vi "Axsun_module.vi"() -> ()   [LabVIEW 2018]
uses:
  cluster_Axsun.ctl
  Queue Manager Actions.ctl
  MessagePacket.ctl
  QueueNames.ctl
  D:/serial sectioning OCT/Axsun laser/AxsunOCTControlConsoleApplicationProject/AxsunOCTControlConsoleApplicationProject/AxsunOCTControl.dll
  AxsunOCTControlConsoleApplicationProject/AxsunOCTControlConsoleApplicationProject/AxsunOCTControl.dll
panel:
  in  "clock delay":u32
  in  "GetStatus":bool
  in  "LaserOnTime":bool
  out "output cluster":T1
  out "GUI error":errorcluster
  in  "Source current OFF":bool
  in  "Source current ON":bool
  in  "stop":bool
  in  "Laser OFF":bool
  in  "Laser ON":bool
  out "processor error":errorcluster
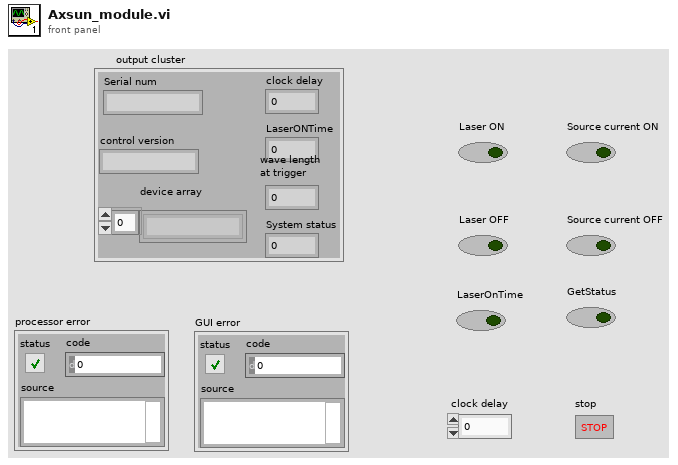
[diagram p1: front panel]
types:
  T1 = typedef "cluster_Axsun.ctl" = cluster{"device array":string[], "control version":string, "Serial num":string, "LaserONTime":i32, "wave length\nat trigger":dbl, "System status":dbl, "clock delay":u32}
  T2 = typedef "MessagePacket.ctl" = cluster{"Message":string, "Parameter":variant}
  T3 = typedef "Queue Manager Actions.ctl" = enum16{"Init", "Enqueue", "Enqueue All", "Preview Queue", "Dequeue", "Get Status", "Flush Queue", "Flush All Queues", "Release All Queues", "Release Queue", "Enqueue at Opposite End"}
  T4 = typedef "QueueNames.ctl" = enum16{"Main GUI", "Main Scan Processor", "Axsun GUI", "Axsun processor", "Main Display", "Main Table Stage GUI", "Main Table Stage Proc.", "Scan Engine", "Vibratome GUI", "Vibratome Processor", "Slice Engine"}
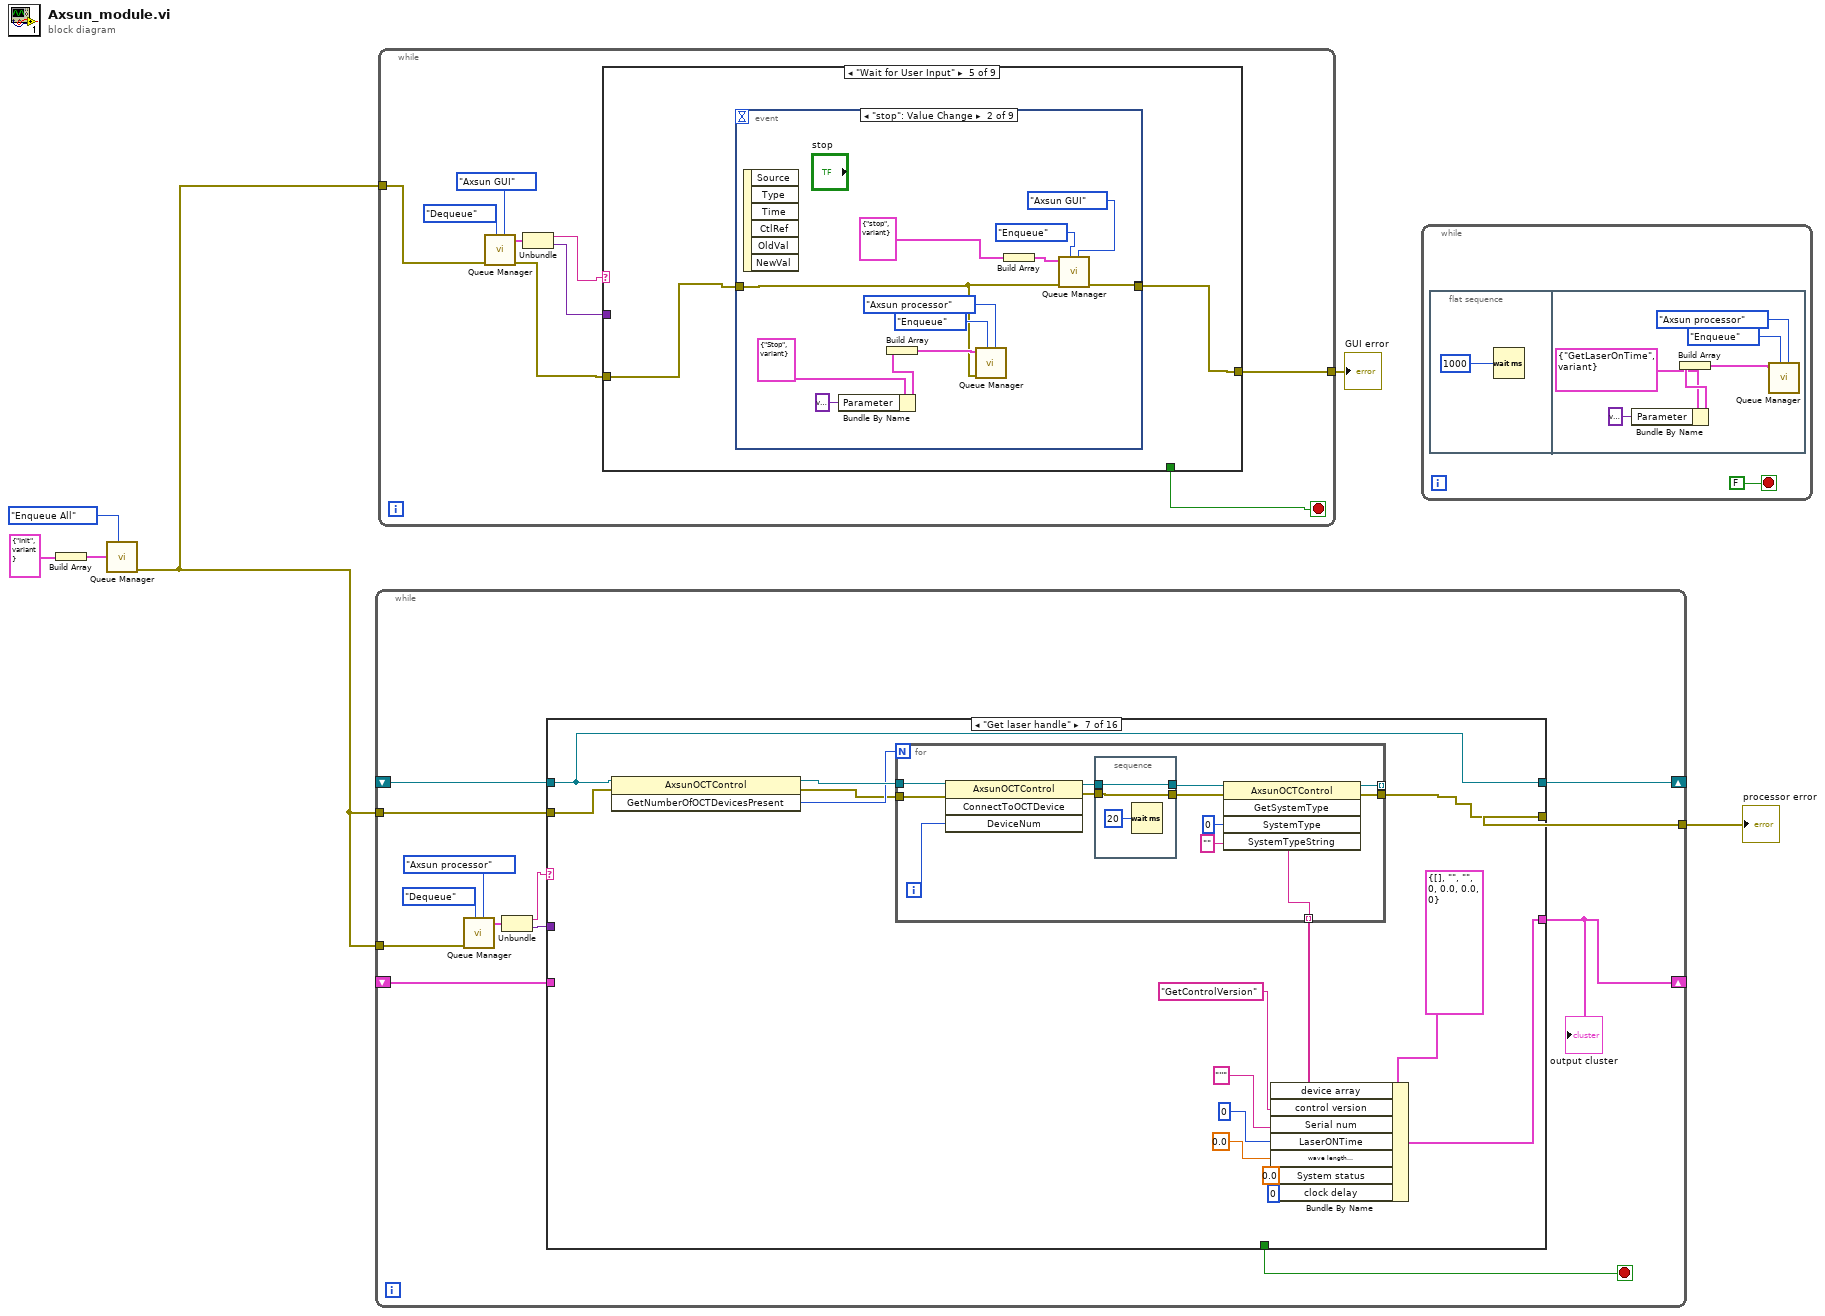
[diagram p0: block diagram]
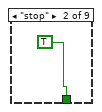
[diagram p3: hidden frame]
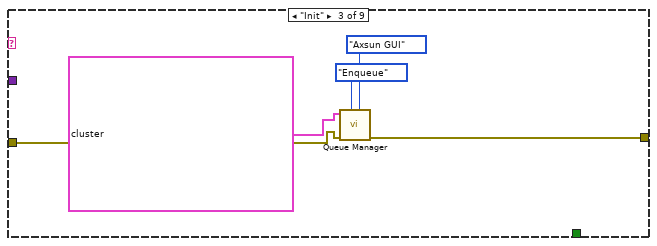
[diagram p4: hidden frame]
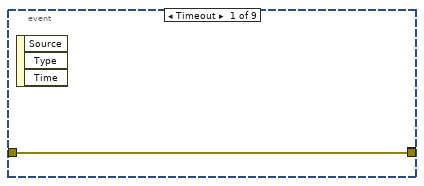
[diagram p6: hidden frame]
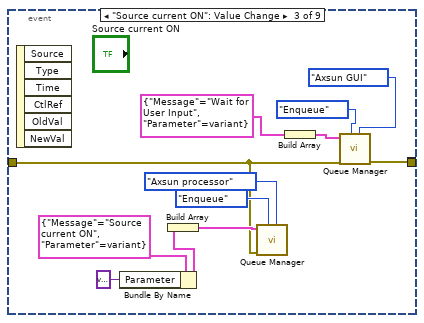
[diagram p7: hidden frame]
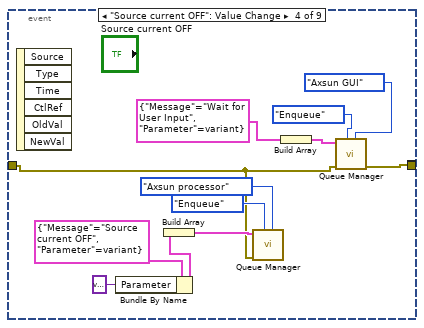
[diagram p8: hidden frame]
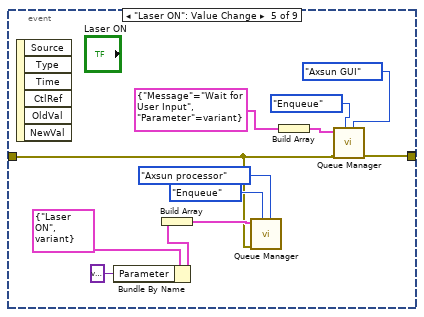
[diagram p9: hidden frame]
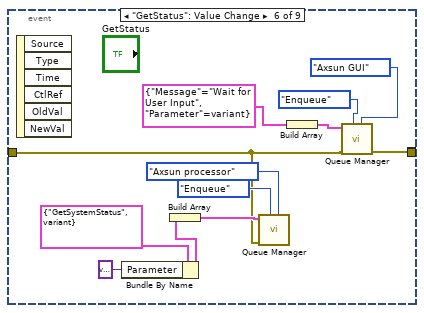
[diagram p10: hidden frame]
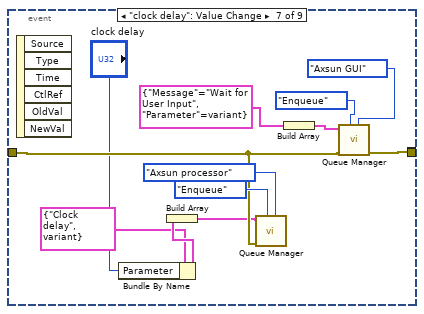
[diagram p11: hidden frame]
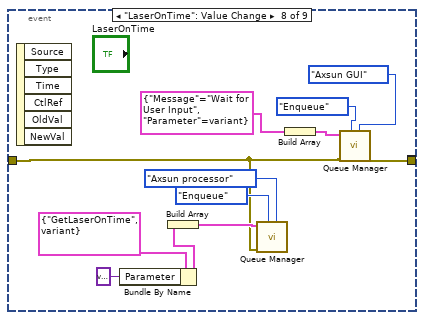
[diagram p12: hidden frame]
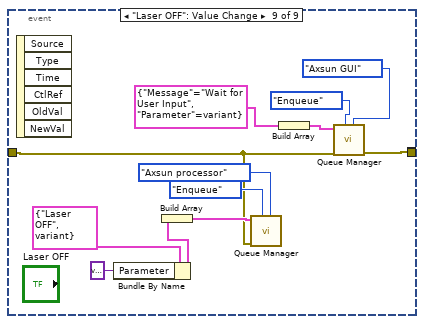
[diagram p13: hidden frame]
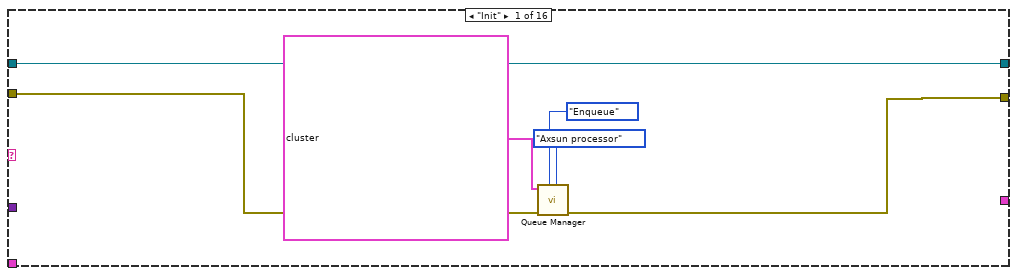
[diagram p18: hidden frame]
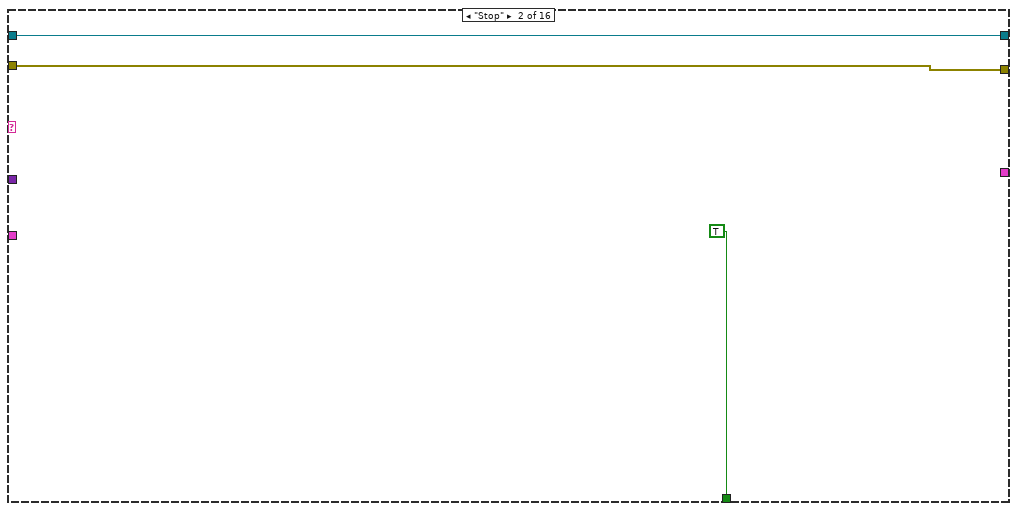
[diagram p19: hidden frame]
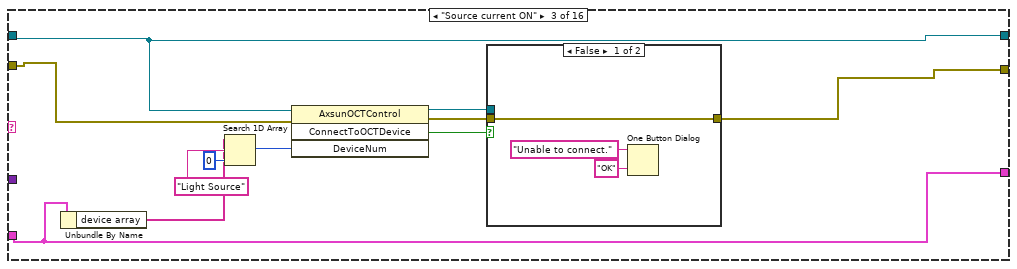
[diagram p20: hidden frame]
diagram:
  n1 = Build Array(T2 {"Message"="Init", "Parameter"=variant} ("Message Packet [In]")) -> (w4:T2[])
  n2 = call "Queue Manager.vi"("Action"=Queue_Manager_Actions."Enqueue All", "Message Packet Array"=w4) -> ("Error Out"=w2:errorcluster)  [unwired: 7 in, 2 out]
  n3 = while {
    shift-right: [w13] -> _
    shift-left: _ -> [w12]
    tunnel: w2 -> [w15]
    shift-right: [w7] -> _
    shift-left: _ -> [w10]
    tunnel: [w9] -> w3
    tunnel: w2 -> [w8]
    stop <- w14 stop-if-true
    n4 = call "Queue Manager.vi"("Queue Name"=QueueNames."Axsun processor", "Action"=Queue_Manager_Actions."Dequeue", "Error In"=w8) -> ("Message Packet [Out]"=w17:T2)  [unwired: 6 in, 2 out]
    n5 = Unbundle(w17) -> ("Message"=w11:string, "Parameter"=w16:variant)
    n6 = case shown="\"Get laser handle\"" w11 {
      tunnel: w16 -> [_ _ _ _ _ _ _ _ _ _ w170 _ _ _ _ _]
      tunnel: w15 -> [w25 w27 w33 w49 w65 w70 w88 w108 w126 w148 w171 w200 w218 w225 w246 _]
      tunnel: [_ TRUE _ _ _ _ _ _ _ _ _ _ _ _ _ _] -> w14
      tunnel: [w20 w26 w31 w48 w64 w67 w83 w106 w127 w146 w167 w198 w216 w226 _ w265] -> w13
      tunnel: w12 -> [w20 w26 w31 w48 w64 w71 w83 w106 w127 w146 w167 w198 w219 w226 w247 _]
      tunnel: [w21 w27 w32 w50 w65 w68 w84 w107 w125 w147 w166 w199 w217 w224 w245 w264] -> w9
      tunnel: [_ _ w30 w47 w63 w66 w76 w105 w124 w144 w164 w197 w214 w220 w241 w263] -> w7
      tunnel: w10 -> [_ _ w30 w47 w63 w66 _ w105 w122 w143 w165 w197 w215 w222 w243 w263]
      frame "Init" {
        n7 = call "Queue Manager.vi"("Queue Name"=QueueNames."Axsun processor", "Action"=Queue_Manager_Actions."Enqueue", "Error In"=w25, "Message Packet Array"=T2[] [{"Message"="Create handle", "Parameter"=variant}, {"Message"="Start Network Control Interface", "Parameter"=variant}, {"Message"="Get laser handle", "Parameter"=variant}, {"Message"="GetControlVersion", "Parameter"=variant}, {"Message"="GetSerialNum", "Parameter"=variant}, {"Message"="GetSystemStatus", "Parameter"=variant}, {"Message"="GetWaveLengthAtSweptTrigger", "Parameter"=variant}, {"Message"="GetLaserOnTime\nGetLaserOnTime", "Parameter"=variant}]) -> ("Error Out"=w21:errorcluster)  [unwired: 5 in, 2 out]
      }
      frame "Stop" {
      }
      frame "Source current ON" {
        n8 = Unbundle By Name(w30) -> ("device array"=w29:string[])
        n9 = Search 1D Array(1D array=w29, element="Light Source", start index (0)=0) -> (index of element=w37:i32)
        n10 = invoke class="AxsunOCTControl" method="ConnectToOCTDevice"(reference=w31, error in=w33, "DeviceNum"=w37) -> (reference out=w36:refnum<k24>, error out=w35:errorcluster, "ConnectToOCTDevice"=w34:bool)  [unwired: 1 in, 1 out]
        n11 = case shown="False" w34 {
          tunnel: w36 -> [_ w45]
          tunnel: w35 -> [w42 w44]
          tunnel: [w42 w43] -> w32
          frame False {
            n12 = One Button Dialog(message="Unable to connect.", button name ("OK")="OK") -> ()  [unwired: 1 out]
          }
          frame True {
            n13 = invoke class="AxsunOCTControl" method="SourceCurrentOn"(reference=w45, error in=w44) -> (error out=w43:errorcluster)  [unwired: 1 in, 2 out]
          }
        }
      }
      frame "Source current OFF" {
        n14 = Unbundle By Name(w47) -> ("device array"=w46:string[])
        n15 = Search 1D Array(1D array=w46, element="Light Source", start index (0)=0) -> (index of element=w54:i32)
        n16 = invoke class="AxsunOCTControl" method="ConnectToOCTDevice"(reference=w48, error in=w49, "DeviceNum"=w54) -> (reference out=w53:refnum<k24>, error out=w52:errorcluster, "ConnectToOCTDevice"=w51:bool)  [unwired: 1 in, 1 out]
        n17 = case shown="True" w51 {
          tunnel: w53 -> [_ w62]
          tunnel: w52 -> [w59 w61]
          tunnel: [w59 w60] -> w50
          frame False {
            n18 = One Button Dialog(message="Unable to connect.", button name ("OK")="OK") -> ()  [unwired: 1 out]
          }
          frame True {
            # "Turn laser emission ON"
            n19 = invoke class="AxsunOCTControl" method="SourceCurrentOff"(reference=w62, error in=w61) -> (error out=w60:errorcluster)  [unwired: 1 in, 2 out]
          }
        }
      }
      frame Default {
      }
      frame "Start Network Control Interface" {
        n20 = invoke class="AxsunOCTControl" method="StartNetworkControlInterface"(reference=w71, error in=w70) -> (reference out=w67:refnum<k24>, error out=w69:errorcluster)  [unwired: 1 in, 1 out]
        n21 = flat-sequence {
          tunnel: w69 -> [w72]
          tunnel: [w72] -> w68
          frame #0 {
            n22 = Wait (ms)(milliseconds to wait=2000) -> ()  [unwired: 1 out]
          }
        }
      }
      frame "Get laser handle" {
        n23 = invoke class="AxsunOCTControl" method="GetNumberOfOCTDevicesPresent"(reference=w83, error in=w88) -> (reference out=w87:refnum<k24>, error out=w85:errorcluster, "GetNumberOfOCTDevicesPresent"=w86:i32)  [unwired: 1 in]
        n24 = for {
          N: w86 -> [_]
          tunnel: w87 -> [w94]
          tunnel: w85 -> [w93]
          tunnel: [w89] -> w78 mode=indexing
          tunnel: [w91] -> w84
          tunnel: [w90] -> _ mode=indexing
          i -> [w92]
          n25 = invoke class="AxsunOCTControl" method="ConnectToOCTDevice"(reference=w94, error in=w93, "DeviceNum"=w92) -> (reference out=w98:refnum<k24>, error out=w97:errorcluster)  [unwired: 1 in, 2 out]
          n26 = stacked-sequence {
            tunnel: w98 -> [w103]
            tunnel: [w103] -> w96
            tunnel: w97 -> [w102]
            tunnel: [w102] -> w95
            frame #0 {
              n27 = Wait (ms)(milliseconds to wait=u32 20) -> ()  [unwired: 1 out]
            }
          }
          n28 = invoke class="AxsunOCTControl" method="GetSystemType"(reference=w96, error in=w95, "SystemType"=u32 0, "SystemTypeString"="") -> (reference out=w90:refnum<k24>, error out=w91:errorcluster, "SystemTypeString"=w89:string)  [unwired: 1 in, 2 out]
        }
        n29 = Bundle By Name(cluster=T1 {"device array"=[], "control version"="", "Serial num"="", "LaserONTime"=0, "wave length\nat trigger"=0.0, "System status"=0.0, "clock delay"=0} ("output cluster"), "device array"=w78, "control version"="GetControlVersion", "Serial num"="''", "LaserONTime"=0, "wave length\nat trigger"=0.0, "System status"=0.0 ("Status"), "clock delay"=u32 0) -> (w76:T1)
      }
      frame "Laser ON" {
        n30 = Unbundle By Name(w105) -> ("device array"=w104:string[])
        n31 = Search 1D Array(1D array=w104, element="Light Source", start index (0)=0) -> (index of element=w112:i32)
        n32 = invoke class="AxsunOCTControl" method="ConnectToOCTDevice"(reference=w106, error in=w108, "DeviceNum"=w112) -> (reference out=w111:refnum<k24>, error out=w110:errorcluster, "ConnectToOCTDevice"=w109:bool)  [unwired: 1 in, 1 out]
        n33 = case shown="True" w109 {
          tunnel: w111 -> [_ w120]
          tunnel: w110 -> [w117 w119]
          tunnel: [w117 w118] -> w107
          frame False {
            n34 = One Button Dialog(message="Unable to .", button name ("OK")="OK") -> ()  [unwired: 1 out]
          }
          frame True {
            # "Turn laser emission ON"
            n35 = invoke class="AxsunOCTControl" method="StartScan"(reference=w120, error in=w119) -> (error out=w118:errorcluster)  [unwired: 1 in, 2 out]
          }
        }
      }
      frame "GetWaveLengthAtSweptTrigger" {
        n36 = Unbundle By Name(w122) -> ("device array"=w121:string[])
        n37 = Search 1D Array(1D array=w121, element="Light Source", start index (0)=0) -> (index of element=w131:i32)
        n38 = invoke class="AxsunOCTControl" method="ConnectToOCTDevice"(reference=w127, error in=w126, "DeviceNum"=w131) -> (reference out=w130:refnum<k24>, error out=w129:errorcluster, "ConnectToOCTDevice"=w128:bool)  [unwired: 1 in, 1 out]
        n39 = case shown="False" w128 {
          tunnel: w130 -> [_ w141]
          tunnel: w129 -> [w136 w140]
          tunnel: [w136 w139] -> w125
          tunnel: [_ w137] -> w123
          frame False {
            n40 = One Button Dialog(message="Unable to .", button name ("OK")="OK") -> ()  [unwired: 1 out]
          }
          frame True {
            # "Turn laser emission ON"
            n41 = invoke class="AxsunOCTControl" method="GetWavelengthAtSweepTrigger"(reference=w141, error in=w140, "Wavelength"=0.0) -> (error out=w139:errorcluster, "Wavelength"=w137:dbl)  [unwired: 1 in, 2 out]
          }
        }
        n42 = Bundle(cluster=w122, "LaserONTime"=w123) -> (w124:T1)  [unwired: 6 in]
      }
      frame "GetLaserOnTime" {
        # "Make active board = laser"
        n43 = Unbundle By Name(w143) -> ("device array"=w142:string[])
        n44 = Search 1D Array(1D array=w142, element="Light Source", start index (0)=0) -> (index of element=w154:i32)
        n45 = invoke class="AxsunOCTControl" method="ConnectToOCTDevice"(reference=w146, error in=w148, "DeviceNum"=w154) -> (reference out=w150:refnum<k24>, error out=w151:errorcluster, "ConnectToOCTDevice"=w149:bool)  [unwired: 1 in, 1 out]
        n46 = case shown="False" w149 {
          tunnel: w151 -> [w157 w161]
          tunnel: w150 -> [_ w162]
          tunnel: [w157 w160] -> w147
          tunnel: [_ w158] -> w145
          frame False {
            n47 = One Button Dialog(message="Unable to connect.", button name ("OK")="OK") -> ()  [unwired: 1 out]
          }
          frame True {
            n48 = invoke class="AxsunOCTControl" method="GetLaserOnTime"(reference=w162, error in=w161, "LaserOnTimeSeconds"=u32 0) -> (error out=w160:errorcluster, "LaserOnTimeSeconds"=w158:u32)  [unwired: 1 in, 2 out]
          }
        }
        n49 = Bundle(cluster=w143, "LaserONTime"=w145) -> (w144:T1)  [unwired: 6 in]
      }
      frame "Clock delay" {
        n50 = Unbundle By Name(w165) -> ("device array"=w172:string[])
        n51 = Search 1D Array(1D array=w172, element="Light Source", start index (0)=0) -> (index of element=w176:i32)
        n52 = invoke class="AxsunOCTControl" method="ConnectToOCTDevice"(reference=w167, error in=w171, "DeviceNum"=w176) -> (reference out=w175:refnum<k24>, error out=w174:errorcluster, "ConnectToOCTDevice"=w173:bool)  [unwired: 1 in, 1 out]
        n53 = case shown="False" w173 {
          tunnel: w175 -> [_ w195]
          tunnel: w174 -> [w189 w191]
          tunnel: [w189 w190] -> w169
          tunnel: w170 -> [_ w194]
          frame False {
            n54 = One Button Dialog(message="Unable to connect.", button name ("OK")="OK") -> ()  [unwired: 1 out]
          }
          frame True {
            n55 = Variant To Data(error in=w191, type=u32 0 ("Delay"), Variant=w194) -> (data=w192:u32)  [unwired: 1 out]
            n56 = invoke class="AxsunOCTControl" method="SetClockDelay"(reference=w195, error in=w191, "Delay"=w192) -> (error out=w190:errorcluster)  [unwired: 1 in, 3 out]
          }
        }
        n57 = case shown="True" TRUE {
          tunnel: w169 -> [w181 w185]
          tunnel: w167 -> [_ w186]
          tunnel: [w181 w184] -> w166
          tunnel: [_ w182] -> w163
          frame False {
            n58 = One Button Dialog(message="Unable to connect.", button name ("OK")="OK") -> ()  [unwired: 1 out]
          }
          frame True {
            n59 = invoke class="AxsunOCTControl" method="GetClockDelay"(reference=w186, error in=w185, "Delay"=u32 0) -> (error out=w184:errorcluster, "Delay"=w182:u32)  [unwired: 1 in, 2 out]
          }
        }
        n60 = Bundle By Name(cluster=w165, "clock delay"=w163) -> (w164:T1)
      }
      frame "Laser OFF" {
        # "Make active board = laser"
        n61 = Unbundle By Name(w197) -> ("device array"=w196:string[])
        n62 = Search 1D Array(1D array=w196, element="Light Source", start index (0)=0) -> (index of element=w204:i32)
        n63 = invoke class="AxsunOCTControl" method="ConnectToOCTDevice"(reference=w198, error in=w200, "DeviceNum"=w204) -> (reference out=w203:refnum<k24>, error out=w202:errorcluster, "ConnectToOCTDevice"=w201:bool)  [unwired: 1 in, 1 out]
        n64 = case shown="True" w201 {
          tunnel: w203 -> [_ w212]
          tunnel: w202 -> [w209 w211]
          tunnel: [w209 w210] -> w199
          frame False {
            n65 = One Button Dialog(message="Unable to connect.", button name ("OK")="OK") -> ()  [unwired: 1 out]
          }
          frame True {
            # "Turn laser emission ON"
            n66 = invoke class="AxsunOCTControl" method="StopScan"(reference=w212, error in=w211) -> (error out=w210:errorcluster)  [unwired: 1 in, 2 out]
          }
        }
      }
      frame "GetControlVersion" {
        n67 = invoke class="AxsunOCTControl" method="GetControlVersion"(reference=w219, error in=w218) -> (reference out=w216:refnum<k24>, error out=w217:errorcluster, "GetControlVersion"=w213:string)  [unwired: 1 in]
        n68 = Bundle By Name(cluster=w215, "control version"=w213) -> (w214:T1)
      }
      frame "GetSerialNum" {
        n69 = Unbundle By Name(w222) -> ("device array"=w223:string[])
        n70 = Search 1D Array(1D array=w223, element="Light Source", start index (0)=0) -> (index of element=w230:i32)
        n71 = invoke class="AxsunOCTControl" method="ConnectToOCTDevice"(reference=w226, error in=w225, "DeviceNum"=w230) -> (reference out=w229:refnum<k24>, error out=w228:errorcluster, "ConnectToOCTDevice"=w227:bool)  [unwired: 1 in, 1 out]
        n72 = case shown="True" w227 {
          tunnel: w229 -> [_ w240]
          tunnel: w228 -> [w235 w239]
          tunnel: [w235 w238] -> w224
          tunnel: [_ w236] -> w221
          frame False {
            n73 = One Button Dialog(message="Unable to connect.", button name ("OK")="OK") -> ()  [unwired: 1 out]
          }
          frame True {
            n74 = invoke class="AxsunOCTControl" method="GetSerialNum"(reference=w240, error in=w239, "SerialNum"="") -> (error out=w238:errorcluster, "SerialNum"=w236:string)  [unwired: 1 in, 2 out]
          }
        }
        n75 = Bundle By Name(cluster=w222, "Serial num"=w221) -> (w220:T1)
      }
      frame "GetSystemStatus" {
        # "Make active board = laser"
        n76 = Unbundle By Name(w243) -> ("device array"=w244:string[])
        n77 = Search 1D Array(1D array=w244, element="Light Source", start index (0)=0) -> (index of element=w253:i32)
        n78 = invoke class="AxsunOCTControl" method="ConnectToOCTDevice"(reference=w247, error in=w246, "DeviceNum"=w253) -> (reference out=w248:refnum<k24>, error out=w249:errorcluster, "ConnectToOCTDevice"=w250:bool)  [unwired: 1 in, 1 out]
        n79 = case shown="True" w250 {
          tunnel: w249 -> [w256 w261]
          tunnel: w248 -> [_ w262]
          tunnel: [w256 w258] -> w245
          tunnel: [_ w257] -> w242
          frame False {
            n80 = One Button Dialog(message="Unable to connect.", button name ("OK")="OK") -> ()  [unwired: 1 out]
          }
          frame True {
            n81 = invoke class="AxsunOCTControl" method="GetSystemStatus"(reference=w262, error in=w261, "StatusArray"=u32[] [], "StatusWordsReturned"=u32 0) -> (error out=w258:errorcluster, "StatusWordsReturned"=w257:u32)  [unwired: 1 in, 3 out]
          }
        }
        n82 = Bundle By Name(cluster=w243, "LaserONTime"=w242) -> (w241:T1)
      }
      frame "Create handle" {
        n83 = constructor class="AxsunOCTControl"() -> (reference out=w265:refnum<k24>, error out=w264:errorcluster)  [unwired: 3 in, 1 out]
      }
    }
    "output cluster" <- w7
  }
  "processor error" <- w3
  n84 = while {
    tunnel: w2 -> [w271]
    tunnel: [w267] -> w1
    stop <- w266 stop-if-true
    n85 = call "Queue Manager.vi"("Queue Name"=QueueNames."Axsun GUI", "Action"=Queue_Manager_Actions."Dequeue", "Error In"=w271) -> ("Error Out"=w268:errorcluster, "Message Packet [Out]"=w272:T2)  [unwired: 6 in, 1 out]
    n86 = Unbundle(w272) -> ("Message"=w270:string, "Parameter"=w269:variant)
    n87 = case shown="\"Wait for User Input\"" w270 {
      tunnel: w269 -> [_ _ _ _ _ _ _ _ _]
      tunnel: w268 -> [w275 _ w281 w282 w284 w382 w383 w384 w385]
      tunnel: [w275 _ w278 w282 w283 w382 w383 w384 w385] -> w267
      tunnel: [_ TRUE _ _ _ _ _ _ _] -> w266
      frame "False", Default {
      }
      frame "stop" {
      }
      frame "Init" {
        n88 = call "Queue Manager.vi"("Queue Name"=QueueNames."Axsun GUI", "Action"=Queue_Manager_Actions."Enqueue", "Error In"=w281, "Message Packet Array"=T2[] [{"Message"="Wait for Complete", "Parameter"=variant}, {"Message"="Set Front Panel", "Parameter"=variant}, {"Message"="Load User Settings", "Parameter"=variant}, {"Message"="Configure Hardware", "Parameter"=variant}, {"Message"="Configure Hardware", "Parameter"=variant}, {"Message"="Wait for User Input", "Parameter"=variant}]) -> ("Error Out"=w278:errorcluster)  [unwired: 5 in, 2 out]
      }
      frame "Set Front Panel" {
      }
      frame "Wait for User Input" {
        n89 = event shown="[1] \"stop\": Value Change" {
          selector: _ -> [_ _ _ _ _ _ _ _ _]
          dyn-events: _ -> [_ _ _ _ _ _ _ _ _]
          timeout: _ -> [_ _ _ _ _ _ _ _ _]
          tunnel: w284 -> [w285 w286 w298 w310 w322 w335 w350 w359 w370]
          tunnel: [_ w287 w299 w311 w326 w334 w349 w358 w372] -> w283
          tunnel: [w285 _ _ _ _ _ _ _ _] -> _
          event Timeout {
            n90 = event-data() -> ()  [unwired: 1 in, 3 out]
          }
          event "stop": Value Change {
            n91 = event-data() -> ()  [unwired: 1 in, 6 out]
            n92 = Bundle By Name(cluster=T2 {"Message"="Stop", "Parameter"=variant} ("Message Packet [In]"), "Parameter"=variant) -> (w293:T2)
            n93 = Build Array(w293) -> (w290:T2[])
            n94 = call "Queue Manager.vi"("Queue Name"=QueueNames."Axsun processor", "Action"=Queue_Manager_Actions."Enqueue", "Error In"=w286, "Message Packet Array"=w290) -> ()  [unwired: 5 in, 3 out]
            n95 = Build Array(T2 {"Message"="stop", "Parameter"=variant} ("Message Packet [In]")) -> (w297:T2[])
            n96 = call "Queue Manager.vi"("Queue Name"=QueueNames."Axsun GUI", "Action"=Queue_Manager_Actions."Enqueue", "Error In"=w286, "Message Packet Array"=w297) -> ("Error Out"=w287:errorcluster)  [unwired: 5 in, 2 out]
          }
          event "Source current ON": Value Change {
            n97 = event-data() -> ()  [unwired: 1 in, 6 out]
            n98 = Bundle By Name(cluster=T2 {"Message"="Source current ON", "Parameter"=variant} ("Message Packet [In]"), "Parameter"=variant) -> (w305:T2)
            n99 = Build Array(w305) -> (w302:T2[])
            n100 = call "Queue Manager.vi"("Queue Name"=QueueNames."Axsun processor", "Action"=Queue_Manager_Actions."Enqueue", "Error In"=w298, "Message Packet Array"=w302) -> ()  [unwired: 5 in, 3 out]
            n101 = Build Array(T2 {"Message"="Wait for User Input", "Parameter"=variant} ("Message Packet [In]")) -> (w309:T2[])
            n102 = call "Queue Manager.vi"("Queue Name"=QueueNames."Axsun GUI", "Action"=Queue_Manager_Actions."Enqueue", "Error In"=w298, "Message Packet Array"=w309) -> ("Error Out"=w299:errorcluster)  [unwired: 5 in, 2 out]
          }
          event "Source current OFF": Value Change {
            n103 = event-data() -> ()  [unwired: 1 in, 6 out]
            n104 = Bundle By Name(cluster=T2 {"Message"="Source current OFF", "Parameter"=variant} ("Message Packet [In]"), "Parameter"=variant) -> (w317:T2)
            n105 = Build Array(w317) -> (w314:T2[])
            n106 = call "Queue Manager.vi"("Queue Name"=QueueNames."Axsun processor", "Action"=Queue_Manager_Actions."Enqueue", "Error In"=w310, "Message Packet Array"=w314) -> ()  [unwired: 5 in, 3 out]
            n107 = Build Array(T2 {"Message"="Wait for User Input", "Parameter"=variant} ("Message Packet [In]")) -> (w321:T2[])
            n108 = call "Queue Manager.vi"("Queue Name"=QueueNames."Axsun GUI", "Action"=Queue_Manager_Actions."Enqueue", "Error In"=w310, "Message Packet Array"=w321) -> ("Error Out"=w311:errorcluster)  [unwired: 5 in, 2 out]
          }
          event "Laser ON": Value Change {
            n109 = event-data() -> ()  [unwired: 1 in, 6 out]
            n110 = Bundle By Name(cluster=T2 {"Message"="Laser ON", "Parameter"=variant} ("Message Packet [In]"), "Parameter"=variant) -> (w329:T2)
            n111 = Build Array(w329) -> (w325:T2[])
            n112 = call "Queue Manager.vi"("Queue Name"=QueueNames."Axsun processor", "Action"=Queue_Manager_Actions."Enqueue", "Error In"=w322, "Message Packet Array"=w325) -> ()  [unwired: 5 in, 3 out]
            n113 = Build Array(T2 {"Message"="Wait for User Input", "Parameter"=variant} ("Message Packet [In]")) -> (w333:T2[])
            n114 = call "Queue Manager.vi"("Queue Name"=QueueNames."Axsun GUI", "Action"=Queue_Manager_Actions."Enqueue", "Error In"=w322, "Message Packet Array"=w333) -> ("Error Out"=w326:errorcluster)  [unwired: 5 in, 2 out]
          }
          event "GetStatus": Value Change {
            n115 = event-data() -> ()  [unwired: 1 in, 6 out]
            n116 = Bundle By Name(cluster=T2 {"Message"="GetSystemStatus", "Parameter"=variant} ("Message Packet [In]"), "Parameter"=variant) -> (w341:T2)
            n117 = Build Array(w341) -> (w338:T2[])
            n118 = call "Queue Manager.vi"("Queue Name"=QueueNames."Axsun processor", "Action"=Queue_Manager_Actions."Enqueue", "Error In"=w335, "Message Packet Array"=w338) -> ()  [unwired: 5 in, 3 out]
            n119 = Build Array(T2 {"Message"="Wait for User Input", "Parameter"=variant} ("Message Packet [In]")) -> (w345:T2[])
            n120 = call "Queue Manager.vi"("Queue Name"=QueueNames."Axsun GUI", "Action"=Queue_Manager_Actions."Enqueue", "Error In"=w335, "Message Packet Array"=w345) -> ("Error Out"=w334:errorcluster)  [unwired: 5 in, 2 out]
          }
          event "clock delay": Value Change {
            n121 = event-data() -> ()  [unwired: 1 in, 6 out]
            n122 = Bundle By Name(cluster=T2 {"Message"="Clock delay", "Parameter"=variant} ("Message Packet [In]"), "Parameter"="clock delay") -> (w353:T2)
            n123 = Build Array(w353) -> (w347:T2[])
            n124 = call "Queue Manager.vi"("Queue Name"=QueueNames."Axsun processor", "Action"=Queue_Manager_Actions."Enqueue", "Error In"=w350, "Message Packet Array"=w347) -> ()  [unwired: 5 in, 3 out]
            n125 = Build Array(T2 {"Message"="Wait for User Input", "Parameter"=variant} ("Message Packet [In]")) -> (w357:T2[])
            n126 = call "Queue Manager.vi"("Queue Name"=QueueNames."Axsun GUI", "Action"=Queue_Manager_Actions."Enqueue", "Error In"=w350, "Message Packet Array"=w357) -> ("Error Out"=w349:errorcluster)  [unwired: 5 in, 2 out]
          }
          event "LaserOnTime": Value Change {
            n127 = event-data() -> ()  [unwired: 1 in, 6 out]
            n128 = Bundle By Name(cluster=T2 {"Message"="GetLaserOnTime", "Parameter"=variant} ("Message Packet [In]"), "Parameter"=variant) -> (w365:T2)
            n129 = Build Array(w365) -> (w362:T2[])
            n130 = call "Queue Manager.vi"("Queue Name"=QueueNames."Axsun processor", "Action"=Queue_Manager_Actions."Enqueue", "Error In"=w359, "Message Packet Array"=w362) -> ()  [unwired: 5 in, 3 out]
            n131 = Build Array(T2 {"Message"="Wait for User Input", "Parameter"=variant} ("Message Packet [In]")) -> (w369:T2[])
            n132 = call "Queue Manager.vi"("Queue Name"=QueueNames."Axsun GUI", "Action"=Queue_Manager_Actions."Enqueue", "Error In"=w359, "Message Packet Array"=w369) -> ("Error Out"=w358:errorcluster)  [unwired: 5 in, 2 out]
          }
          event "Laser OFF": Value Change {
            n133 = event-data() -> ()  [unwired: 1 in, 6 out]
            n134 = Bundle By Name(cluster=T2 {"Message"="Laser OFF", "Parameter"=variant} ("Message Packet [In]"), "Parameter"=variant) -> (w377:T2)
            n135 = Build Array(w377) -> (w374:T2[])
            n136 = call "Queue Manager.vi"("Queue Name"=QueueNames."Axsun processor", "Action"=Queue_Manager_Actions."Enqueue", "Error In"=w370, "Message Packet Array"=w374) -> ()  [unwired: 5 in, 3 out]
            n137 = Build Array(T2 {"Message"="Wait for User Input", "Parameter"=variant} ("Message Packet [In]")) -> (w381:T2[])
            n138 = call "Queue Manager.vi"("Queue Name"=QueueNames."Axsun GUI", "Action"=Queue_Manager_Actions."Enqueue", "Error In"=w370, "Message Packet Array"=w381) -> ("Error Out"=w372:errorcluster)  [unwired: 5 in, 2 out]
          }
        }
      }
      frame "Wait for Complete" {
      }
      frame "Configure Hardware" {
      }
      frame "Load User Settings" {
      }
      frame "Init Variables" {
      }
    }
  }
  "GUI error" <- w1
  n139 = while {
    stop <- FALSE stop-if-true
    n140 = flat-sequence {
      frame #0 {
        n141 = Wait (ms)(milliseconds to wait=u32 1000) -> ()  [unwired: 1 out]
      }
      frame #1 {
        n142 = Bundle By Name(cluster=T2 {"Message"="GetLaserOnTime", "Parameter"=variant} ("Message Packet [In]"), "Parameter"=variant) -> (w393:T2)
        n143 = Build Array(w393) -> (w391:T2[])
        n144 = call "Queue Manager.vi"("Queue Name"=QueueNames."Axsun processor", "Action"=Queue_Manager_Actions."Enqueue", "Message Packet Array"=w391) -> ()  [unwired: 6 in, 3 out]
      }
    }
  }
